vi "Tosca-TCP test (stay open).vi"() -> ()   [LabVIEW 2020]
panel:
  out "result":i32
  in  "Close Button":bool
  in  "Open Button":bool
  in  "stop":bool
  in  "Send Button":bool
  out "date/time":string
  in  "command":string="Time"
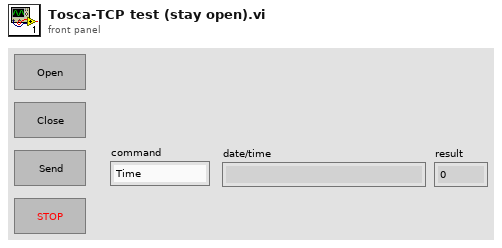
[diagram p1: front panel]
types:
  T1 = enum16{"Standard", "Buffered", "CRLF", "Immediate"}
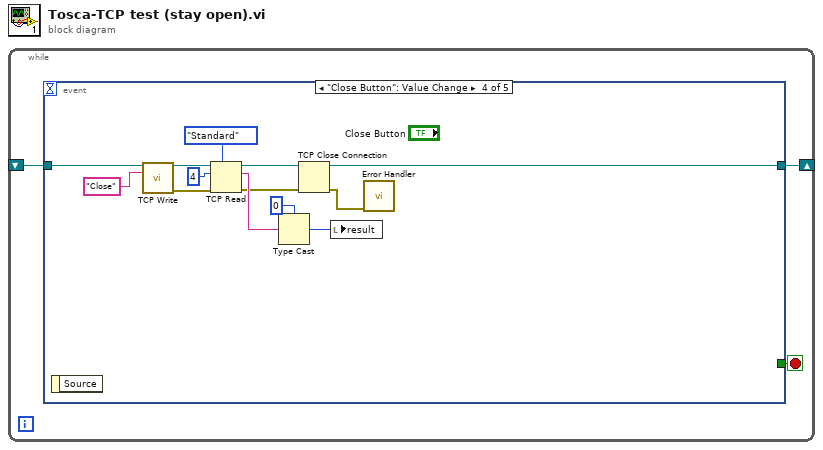
[diagram p0: block diagram]
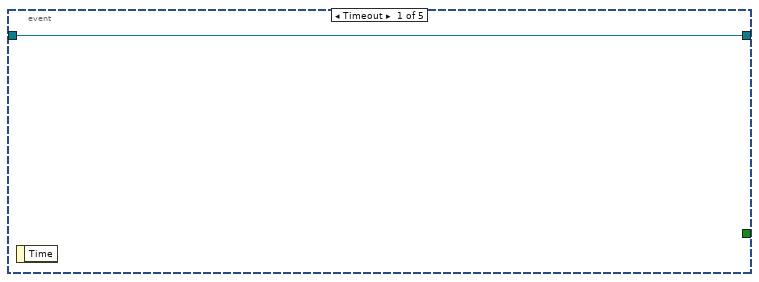
[diagram p2: hidden frame]
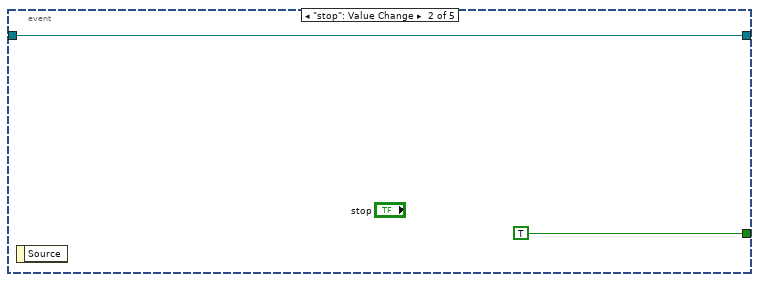
[diagram p3: hidden frame]
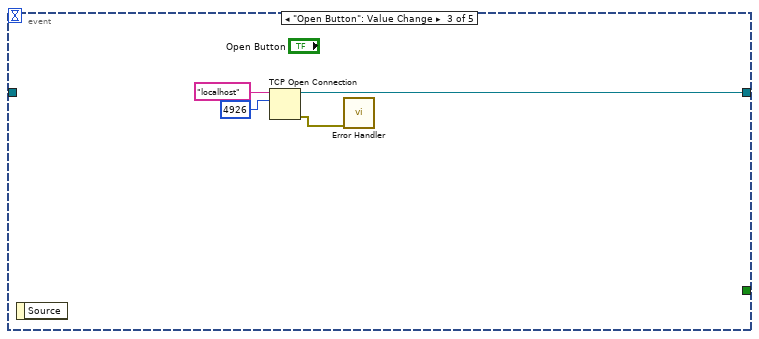
[diagram p4: hidden frame]
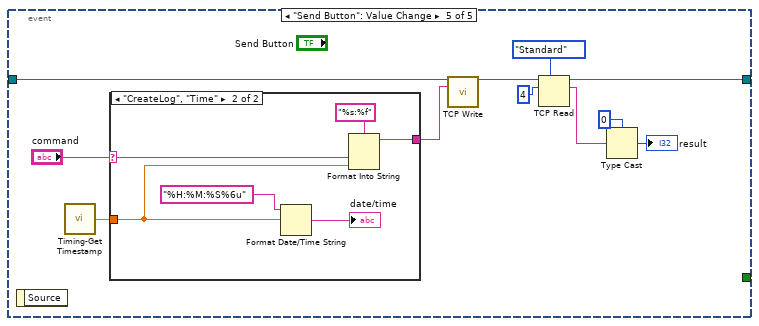
[diagram p5: hidden frame]
diagram:
  n1 = while {
    shift-right: [w2] -> _
    shift-left: _ -> [w1]
    stop <- w3 stop-if-true
    n2 = event shown="[3] \"Close Button\": Value Change" {
      selector: _ -> [_ _ _ _ _]
      dyn-events: _ -> [_ _ _ _ _]
      timeout: _ -> [_ _ _ _ _]
      tunnel: [_ TRUE _ _ _] -> w3
      tunnel: [w4 w5 w8 w23 w29] -> w2
      tunnel: w1 -> [w4 w5 _ w16 w33]
      event Timeout {
        n3 = event-data() -> ()  [unwired: 1 in, 1 out]
      }
      event "stop": Value Change {
        n4 = event-data() -> ()  [unwired: 1 in, 1 out]
      }
      event "Open Button": Value Change {
        n5 = event-data() -> ()  [unwired: 1 in, 1 out]
        n6 = TCP Open Connection(address="localhost", remote port or service name=u16 4926) -> (connection ID=w8:refnum<k5>, error out=w7:errorcluster)  [unwired: 3 in]
        n7 = call "Error Handler.vi"("error in (no error)"=w7) -> ()  [unwired: 13 in, 2 out]
      }
      event "Close Button": Value Change {
        n8 = event-data() -> ()  [unwired: 1 in, 1 out]
        n9 = call "TCP Write.vi"("connection ID"=w16, "data string"="Close") -> ("connection ID out"=w19:refnum<k5>, "error out"=w12:errorcluster)  [unwired: 11 in, 1 out]
        n10 = TCP Read(connection ID=w19, bytes to read=4, error in (no error)=w12, 7:T1."Standard" ("mode (standard)")) -> (connection ID out=w14:refnum<k5>, data out=w17:string, error out=w11:errorcluster)  [unwired: 1 in]
        n11 = Type Cast(type=0, x=w17) -> (*(type *) &x=w13:i32)
        n12 = TCP Close Connection(connection ID=w14, error in (no error)=w11) -> (connection ID out=w23:refnum<k5>, error out=w22:errorcluster)  [unwired: 1 in]
        n13 = local write "result"(w13) -> ()
        n14 = call "Error Handler.vi"("error in (no error)"=w22) -> ()  [unwired: 13 in, 2 out]
      }
      event "Send Button": Value Change {
        n15 = event-data() -> ()  [unwired: 1 in, 1 out]
        n16 = call "Timing-Get Timestamp.vi"() -> ("double precision float"=w24:dbl)  [unwired: 14 in, 1 out]
        n17 = case shown="\"CreateLog\", \"Time\"" "command" {
          selector: "command" -> [w35 w38]
          tunnel: [w35 w37] -> w25
          tunnel: w24 -> [_ w36]
          frame "", Default {
          }
          frame "CreateLog", "Time" {
            n18 = Format Date/Time String(time format string (%c)="%H:%M:%S%6u", seconds (now)=w36) -> (date/time string=→"date/time":string)  [unwired: 1 in]
            n19 = Format Into String(format string="%s:%f", w38, w36) -> (resulting string=w37:string)  [unwired: 2 in, 1 out]
          }
        }
        n20 = call "TCP Write.vi"("connection ID"=w33, "data string"=w25) -> ("connection ID out"=w30:refnum<k5>)  [unwired: 11 in, 2 out]
        n21 = TCP Read(connection ID=w30, bytes to read=4, 7:T1."Standard" ("mode (standard)")) -> (connection ID out=w29:refnum<k5>, data out=w27:string)  [unwired: 2 in, 1 out]
        n22 = Type Cast(type=0, x=w27) -> (*(type *) &x=→"result":i32)
      }
    }
  }
